vi "Adapt Data to chart new v02.vi"(10 "1D Array":T1(array[cluster]), 11 "Waveform Graph":cluster{dbl, dbl, dbl}[][](array[cluster])=[[{1.0, 1.0, 1.0}, {1.0, 1.0, 1.0}, {1.0, 1.0, 1.0}], [{2.0, 2.0, 2.0}, {2.0, 2.0, 2.0}, {0.0, 0.0, 0.0}], [{3.0, 3.0, 3.0}, {0.0, 0.0, 0.0}, {0.0, 0.0, 0.0}]]) -> (2 "PlotNames":string[](array[string]), 3 "Data":dbl[][](graph) caption="Waveform Chart - dark")   [LabVIEW 2016]
uses:
  <userlib>/_OpenG.lib/array/array.llb/Conditional Auto-Indexing Tunnel (String)__ogtk.vi
  <userlib>/_OpenG.lib/array/array.llb/Filter 1D Array with Scalar (String)__ogtk.vi
  <userlib>/_OpenG.lib/array/array.llb/Conditional Auto-Indexing Tunnel (DBL)__ogtk.vi
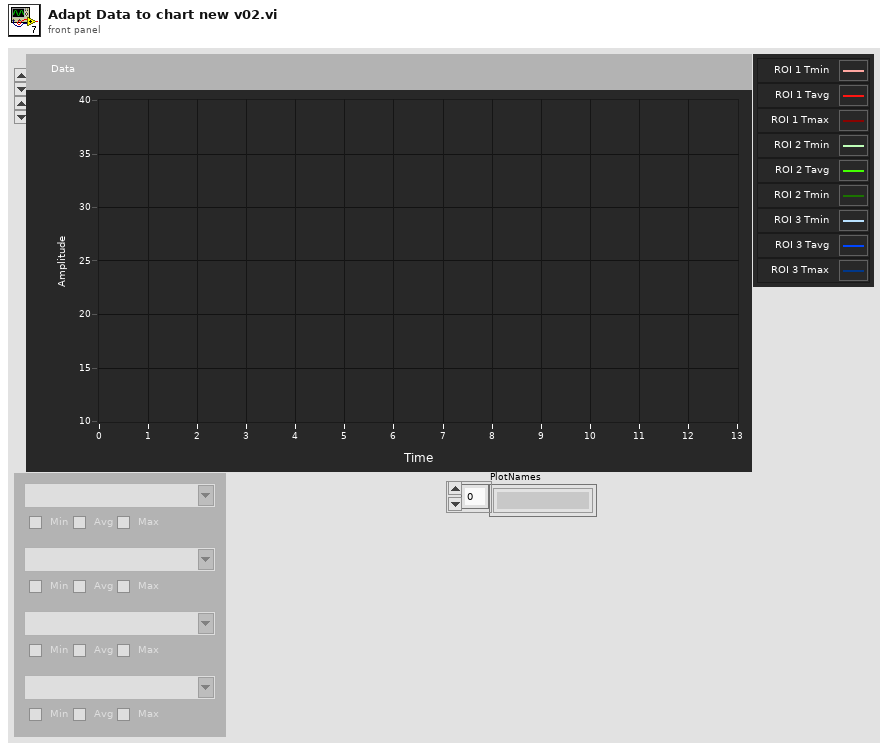
[diagram p1: front panel]
types:
  T1 = cluster{"Combo Box":string, "Option":cluster{"Min":bool, "Avg":bool, "Max":bool}}[]
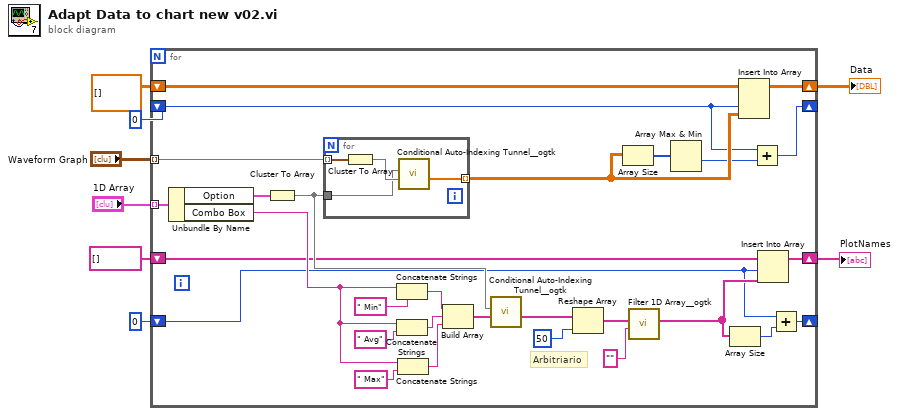
[diagram p0: block diagram]
diagram:
  n1 = for {
    tunnel: "Waveform Graph" -> [w37] mode=indexing
    shift-right: [w35] -> w6
    shift-left: dbl[][] [] ("Filtered Array out") -> [w36]
    shift-right: [w31] -> _
    shift-left: 0 -> [w30]
    tunnel: "1D Array" -> [w29] mode=indexing
    shift-right: [w14] -> w2
    shift-left: string[] [] ("filtered array") -> [w13]
    shift-right: [w10] -> _
    shift-left: 0 -> [w9]
    # "Arbitriario"
    n2 = Unbundle By Name(w29) -> ("Option"=w28:cluster{"Min":bool, "Avg":bool, "Max":bool}, "Combo Box"=w17:string)
    n3 = Cluster To Array(cluster=w28) -> (array=w16:bool[])
    n4 = for {
      tunnel: w37 -> [w41] mode=indexing
      tunnel: [w39] -> w34 mode=indexing
      tunnel: w16 -> [w38]
      n5 = Cluster To Array(cluster=w41) -> (array=w40:dbl[])
      n6 = call-poly <userlib>:"Conditional Auto-Indexing Tunnel__ogtk.vi"("Array in"=w40, "Elements to keep"=w38) -> ("Filtered Array out"=w39:dbl[])  [unwired: 5 in]
    }
    n7 = Concatenate Strings(w17, " Min") -> (w21:string)
    n8 = Concatenate Strings(w17, " Avg") -> (w20:string)
    n9 = Concatenate Strings(w17, " Max") -> (w19:string)
    n10 = Build Array(w21, w20, w19) -> (w18:string[])
    n11 = call-poly <userlib>:"Conditional Auto-Indexing Tunnel__ogtk.vi"("Array in"=w18, "Elements to keep"=w16) -> ("Filtered Array out"=w15:string[])  [unwired: 5 in]
    n12 = Reshape Array(w15, 50 ("dimension size")) -> (w27:string[])
    n13 = Array Size(array=w34) -> (size(s)=w33:i32[])
    n14 = call-poly <userlib>:"Filter 1D Array__ogtk.vi"("items to filter"="", "array"=w27) -> ("filtered array"=w12:string[])  [unwired: 4 in, 1 out]
    n15 = Array Max & Min(array=w33) -> (min value=w32:i32)  [unwired: 3 out]
    n16 = Array Size(array=w12) -> (size(s)=w11:i32)
    n17 = Insert Into Array(array=w36, index (col)=w30, new element=w34) -> (w35:dbl[][])  [unwired: 1 in]
    n18 = Add(x=w30, y=w32) -> (x+y=w31:i32)
    n19 = Insert Into Array(array=w13, index=w9, new element=w12) -> (w14:string[])
    n20 = Add(x=w9, y=w11) -> (x+y=w10:i32)
  }
  "Data" <- w6
  "PlotNames" <- w2
